vi "S1-S2-SenseBall.vi"(8 "Ball in Process in":bool, 11 "Sense Ball":bool) -> (0 "Ball Counter":dbl, 3 "Ball in Process out":bool)   [LabVIEW 2011]
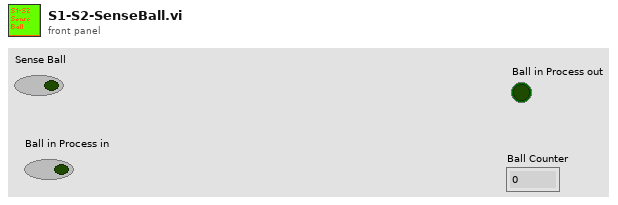
[diagram p1: front panel]
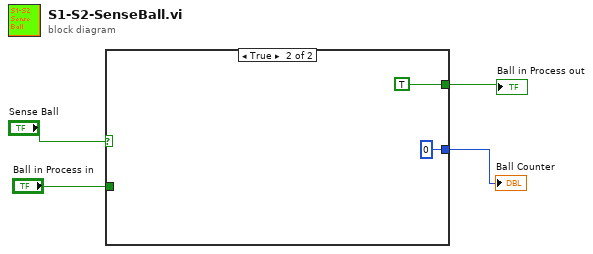
[diagram p0: block diagram]
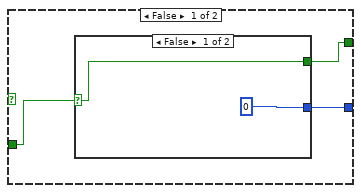
[diagram p2: hidden frame]
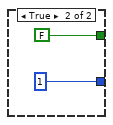
[diagram p3: hidden frame]
diagram:
  n1 = case shown="True" "Sense Ball" {
    tunnel: [w5 TRUE] -> w3
    tunnel: "Ball in Process in" -> [w7 _]
    tunnel: [w6 0] -> w1
    frame False {
      n2 = case shown="False" w7 {
        selector: w7 -> [w9 _]
        tunnel: [0 1] -> w6
        tunnel: [w9 FALSE] -> w5
        frame False {
        }
        frame True {
        }
      }
    }
    frame True {
    }
  }
  "Ball in Process out" <- w3
  "Ball Counter" <- w1
